vi "Demo Navigation Bar More.vi"(8 "error in (no error)":errorcluster) -> (0 "error out":errorcluster)   [LabVIEW 2011]
uses:
  VIremote.llb/VIremoteEvent.ctl
  VIremote.llb/VIremoteBarButton.ctl
  VIremote.llb/VIremoteFunction.ctl
  VIremote.llb/VIremoteStatus.ctl
  VIremote.llb/VIremoteNavigationBar.ctl
panel:
  in  "Tap to change button 3 color":u32(colorbox)=16777216 caption="Prior to iOS 5 you can't\nchange color."
  in  "Clear history":bool
  in  "Show/Hide Prompt":bool caption="Prompt"
  in  "Show/Hide Other Buttons":bool caption="Other Buttons"
  in  "Button 3":T1
  out "Last button tap":string
  in  "Button 2":T1
  in  "Show/Hide Backbutton":bool=TRUE caption="Back Button"
  in  "Back Button Text":string="Navigation Bar"
  in  "Show/Hide Bar":bool=TRUE caption="Bar"
  in  "Button 1":T1
  in  "Tap to change bar color":u32(colorbox)=12227415 caption="Transparent = default blue"
  in  "VIremoteEvent":T2=enum."Connection Closed"
  # "Show"
  # "Show"
  # "Show"
  # "Hide"
  # "Hide"
  # "Hide"
  # "Tap a numeric control to bring up the numeric keyboard.\nThis control has been customized with bigger up/down buttons so they are easier to hit."
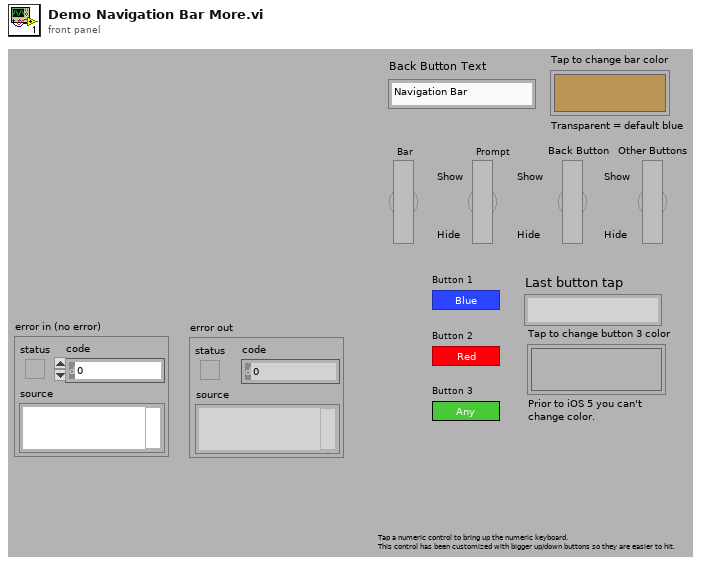
[diagram p1: front panel]
types:
  T1 = typedef "VIremoteBarButton.ctl" = bool
  T2 = typedef "VIremoteEvent.ctl" = enum16{"No Event", "Connection Closed", "Navigate Back", "Enter Background", "Enter Foreground", "Portrait", "Portrait Upside Down", "Landscape Left", "Landscape Right"}
  T3 = typedef "VIremoteFunction.ctl" = enum16{"Do nothing", "Stop controller", "Close this connection", "Show info panel", "Set VI to control", "Set Accelerometer freq (Hz)", "Show Alert message", "Start Sound Input", "Stop Sound Input", "Set Volume (0-100)", "Set sound output Speaker", "Set sound output Receiver", "Play Sound", "Repeat Sound", "Stop Sound", "Pause Sound", "Resume Sound", "Set panel width of caller (320 or 480)", "Set Panel Size to Portrait", "Set Panel Size to Landscape", "Set Panel Size as Current Orientation", "Allow all UI Orientations", "Send user notification", "Disable Scrolling", "Normal Scrolling", "Page Scrolling", "Set Scroll Offset", "Page Indicator Position"}
  T4 = typedef "VIremoteStatus.ctl" = enum16{"Connected BOOL", "Number of connections DBL", "VIremoteController ver.", "VIremote ver. DBL", "Screen width DBL", "Screen height DBL", "Current navigation bar height DBL", "Current UI orientation", "Background supported BOOL", "Background state BOOL", "Device UI idiom (0=phone,1=iPad) DBL", "Device name", "Device unique id", "Device system ver.", "Device model", "Device HW model"}
  T5 = enum8{"Enabled", "Disabled", "Disabled and Grayed Out"}
  T6 = typedef "VIremoteNavigationBar.ctl" = enum16{"Show Bar", "Hide Bar", "Clear History", "Set Bar Tint Color", "Set Bar Title", "Set Bar Prompt", "Show Back Button", "Hide Back Button", "Set Back Button Text", "Add Right Button", "Add Left Button", "Remove Button"}
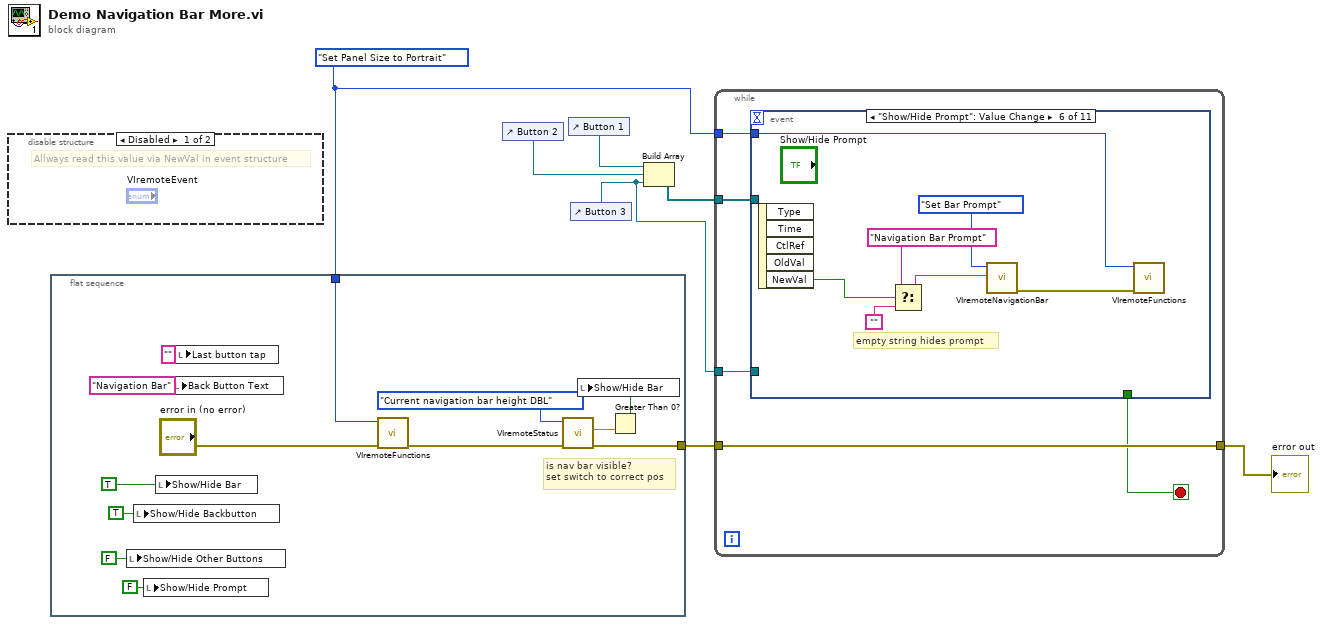
[diagram p0: block diagram]
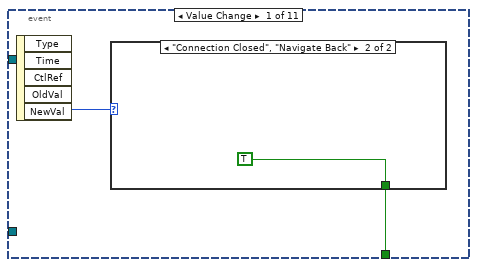
[diagram p3: hidden frame]
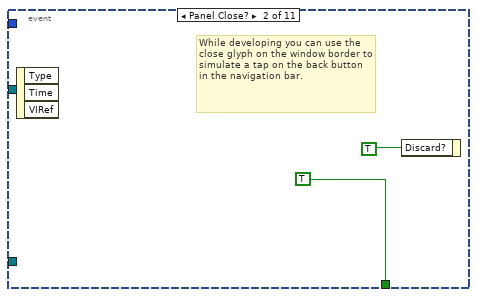
[diagram p5: hidden frame]
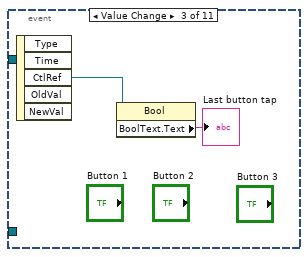
[diagram p6: hidden frame]
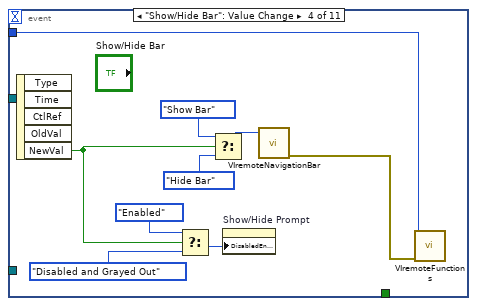
[diagram p7: hidden frame]
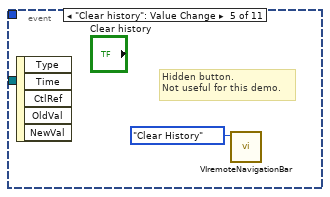
[diagram p8: hidden frame]
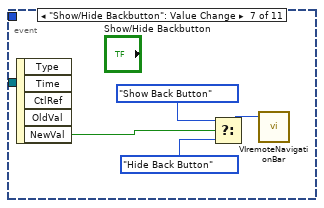
[diagram p9: hidden frame]
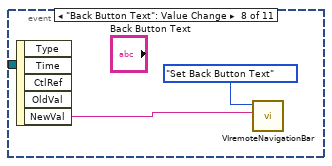
[diagram p10: hidden frame]
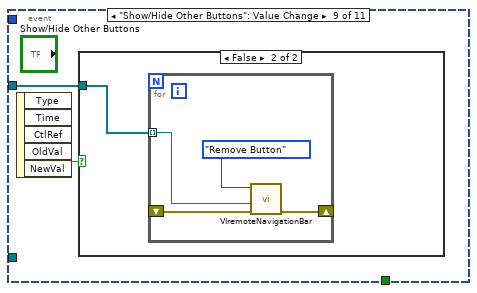
[diagram p11: hidden frame]
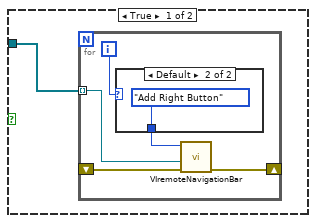
[diagram p12: hidden frame]
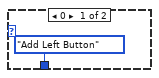
[diagram p13: hidden frame]
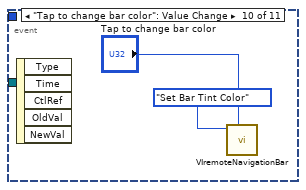
[diagram p14: hidden frame]
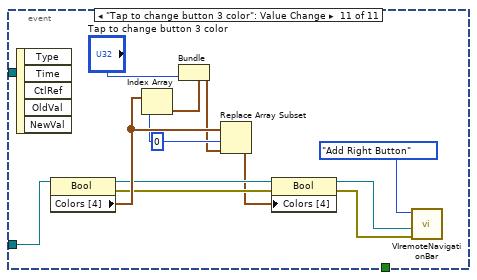
[diagram p15: hidden frame]
diagram:
  w3 = VIremoteFunction."Set Panel Size to Portrait" ("Function")
  n1 = disable-structure shown="Disabled" {
    frame Disabled {
      # "Allways read this value via NewVal in event structure"
    }
    frame Enabled {
    }
  }
  n2 = flat-sequence {
    tunnel: [w18] -> w7
    tunnel: w3 -> [w17]
    frame #0 {
      # "is nav bar visible?\nset switch to correct pos"
      n3 = local write "Show/Hide Other Buttons"(FALSE ("Show/Hide Prompt")) -> ()
      n4 = local write "Show/Hide Backbutton"(TRUE ("Show/Hide Prompt")) -> ()
      n5 = local write "Show/Hide Prompt"(FALSE ("Show/Hide Prompt")) -> ()
      n6 = local write "Show/Hide Bar"(TRUE ("Show/Hide Prompt")) -> ()
      n7 = local write "Back Button Text"("Navigation Bar" ("Back Button Text")) -> ()
      n8 = local write "Last button tap"("" ("Last button tap")) -> ()
      n9 = call "VIremoteFunctions.vi"("error in (no error)"="error in (no error)", "Function"=w17) -> ("error out"=w19:errorcluster)  [unwired: 4 in, 5 out]
      n10 = call "VIremoteStatus.vi"("error in (no error)"=w19, "Status item"=VIremoteStatus."Current navigation bar height DBL") -> ("error out"=w18:errorcluster, "DBL"=w16:dbl)  [unwired: 1 in, 7 out]
      n11 = Greater Than 0?(x=w16) -> (x > 0?=w15:bool)
      n12 = local write "Show/Hide Bar"(w15) -> ()
    }
  }
  n13 = control-ref of="Button 2"() -> (w5:refnum<vi>)
  n14 = control-ref of="Button 1"() -> (w6:refnum<vi>)
  n15 = control-ref of="Button 3"() -> (w1:refnum<vi>)
  n16 = Build Array(w6, w5, w1) -> (w4:refnum<vi>[])
  n17 = while {
    tunnel: [w25] -> w2
    tunnel: w7 -> [w25]
    tunnel: w4 -> [w23]
    tunnel: w3 -> [w22]
    tunnel: w1 -> [w21]
    stop <- w24 stop-if-true
    n18 = event shown="[5] \"Show/Hide Prompt\": Value Change" {
      selector: _ -> [_ _ _ _ _ _ _ _ _ _ _]
      dyn-events: _ -> [_ _ _ _ _ _ _ _ _ _ _]
      timeout: _ -> [_ _ _ _ _ _ _ _ _ _ _]
      tunnel: [w26 TRUE ("Discard?") _ _ _ _ _ _ _ _ _] -> w24
      tunnel: w23 -> [_ _ _ _ _ _ _ _ w56 _ _]
      tunnel: w22 -> [_ _ _ w37 _ w43 _ _ _ _ _]
      tunnel: w21 -> [_ _ _ _ _ _ _ _ _ _ w83]
      event Value Change {
        n19 = event-data() -> ("NewVal"=w27:T2)  [unwired: 5 out]
        n20 = case shown="\"Connection Closed\", \"Navigate Back\"" w27 {
          tunnel: [_ TRUE] -> w26
          frame "No Event", Default {
          }
          frame "Connection Closed", "Navigate Back" {
          }
        }
      }
      event Panel Close? {
        # "While developing you can use the close glyph on the window border to simulate a tap on the back button in the navigation bar."
        n21 = event-data() -> ()  [unwired: 4 out]
        n22 = event-data("Discard?"=TRUE) -> ()  [unwired: 1 in, 1 out]
      }
      event Value Change {
        n23 = event-data() -> ("CtlRef"=w32:refnum<vi>)  [unwired: 5 out]
        n24 = property class="Bool"(reference=w32) -> ("BoolText.Text"=→"Last button tap":string)  [unwired: 1 in, 2 out]
      }
      event "Show/Hide Bar": Value Change {
        n25 = event-data() -> ("NewVal"=w35:bool)  [unwired: 5 out]
        n26 = Select(t=T5."Enabled" ("Disabled"), s=w35, f=T5."Disabled and Grayed Out" ("Disabled")) -> (s? t:f=w36:T5)
        n27 = Select(t=VIremoteNavigationBar."Show Bar" ("Func"), s=w35, f=VIremoteNavigationBar."Hide Bar" ("Func")) -> (s? t:f=w39:T6)
        n28 = property on="Show/Hide Prompt" class="Bool (strict)"("DisabledEnum"=w36) -> ()  [unwired: 2 in, 2 out]
        n29 = call "VIremoteNavigationBar.vi"("Func"=w39) -> ("error out"=w38:errorcluster)  [unwired: 4 in, 6 out]
        n30 = call "VIremoteFunctions.vi"("error in (no error)"=w38, "Function"=w37) -> ()  [unwired: 4 in, 6 out]
      }
      event "Clear history": Value Change {
        # "Hidden button.\nNot useful for this demo."
        n31 = event-data() -> ()  [unwired: 6 out]
        n32 = call "VIremoteNavigationBar.vi"("Func"=VIremoteNavigationBar."Clear History") -> ()  [unwired: 4 in, 7 out]
      }
      event "Show/Hide Prompt": Value Change {
        # "empty string hides prompt"
        n33 = event-data() -> ("NewVal"=w48:bool)  [unwired: 5 out]
        n34 = Select(t="Navigation Bar Prompt" ("String"), s=w48, f="") -> (s? t:f=w46:string)
        n35 = call "VIremoteNavigationBar.vi"("String (\"\")"=w46, "Func"=VIremoteNavigationBar."Set Bar Prompt") -> ("error out"=w44:errorcluster)  [unwired: 3 in, 6 out]
        n36 = call "VIremoteFunctions.vi"("error in (no error)"=w44, "Function"=w43) -> ()  [unwired: 4 in, 6 out]
      }
      event "Show/Hide Backbutton": Value Change {
        n37 = event-data() -> ("NewVal"=w53:bool)  [unwired: 5 out]
        n38 = Select(t=VIremoteNavigationBar."Show Back Button" ("Func"), s=w53, f=VIremoteNavigationBar."Hide Back Button" ("Func")) -> (s? t:f=w50:T6)
        n39 = call "VIremoteNavigationBar.vi"("Func"=w50) -> ()  [unwired: 4 in, 7 out]
      }
      event "Back Button Text": Value Change {
        n40 = event-data() -> ("NewVal"=w54:string)  [unwired: 5 out]
        n41 = call "VIremoteNavigationBar.vi"("String (\"\")"=w54, "Func"=VIremoteNavigationBar."Set Back Button Text") -> ()  [unwired: 3 in, 7 out]
      }
      event "Show/Hide Other Buttons": Value Change {
        n42 = event-data() -> ("NewVal"=w57:bool)  [unwired: 5 out]
        n43 = case shown="False" w57 {
          tunnel: w56 -> [w58 w66]
          frame True {
            n44 = for {
              shift-right: [w62] -> _
              shift-left: _ -> [w61]
              tunnel: w58 -> [w60] mode=indexing
              i -> [w59]
              n45 = case shown="Default" w59 {
                tunnel: [VIremoteNavigationBar."Add Left Button" ("Func") VIremoteNavigationBar."Add Right Button" ("Func")] -> w63
                frame 0 {
                }
                frame Default {
                }
              }
              n46 = call "VIremoteNavigationBar.vi"("error in (no error)"=w61, "Button reference"=w60, "Func"=w63) -> ("error out"=w62:errorcluster)  [unwired: 2 in, 6 out]
            }
          }
          frame False {
            n47 = for {
              shift-right: [w69] -> _
              shift-left: _ -> [w68]
              tunnel: w66 -> [w67] mode=indexing
              n48 = call "VIremoteNavigationBar.vi"("error in (no error)"=w68, "Button reference"=w67, "Func"=VIremoteNavigationBar."Remove Button") -> ("error out"=w69:errorcluster)  [unwired: 2 in, 6 out]
            }
          }
        }
      }
      event "Tap to change bar color": Value Change {
        n49 = event-data() -> ()  [unwired: 6 out]
        n50 = call "VIremoteNavigationBar.vi"("Color"="Tap to change bar color", "Func"=VIremoteNavigationBar."Set Bar Tint Color") -> ()  [unwired: 3 in, 7 out]
      }
      event "Tap to change button 3 color": Value Change {
        w81 = 0 ("index")
        n51 = event-data() -> ()  [unwired: 6 out]
        n52 = property class="Bool"(reference=w83) -> (reference out=w76:refnum<vi>, error out=w77:errorcluster, "Colors [4]"=w82:cluster{u32, u32}[])  [unwired: 1 in]
        n53 = Index Array(array=w82, index=w81) -> (element=w80:cluster{u32, u32})
        n54 = Bundle(cluster=w80, "Tap to change button 3 color") -> (w78:cluster{u32, u32})  [unwired: 1 out]
        n55 = Replace Array Subset(array=w82, new element=w78, index=w81) -> (w73:cluster{u32, u32}[])
        n56 = property class="Bool"(reference=w76, error in=w77, "Colors [4]"=w73) -> (reference out=w74:refnum<vi>, error out=w75:errorcluster)
        n57 = call "VIremoteNavigationBar.vi"("error in (no error)"=w75, "Button reference"=w74, "Func"=VIremoteNavigationBar."Add Right Button") -> ()  [unwired: 2 in, 7 out]
      }
    }
  }
  "error out" <- w2
